vi "subvi_slope.vi"(1 "X1":dbl, 2 "X2":dbl, 3 "Y1":dbl, 4 "Y2":dbl) -> (0 "SLOPE":dbl)   [LabVIEW 2023]
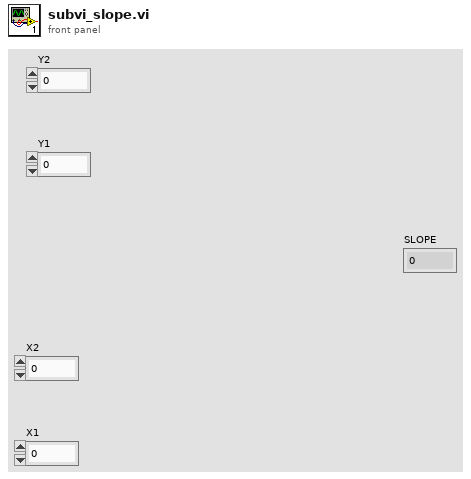
[diagram p1: front panel]
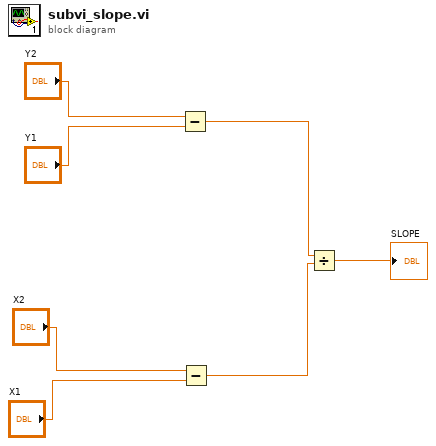
[diagram p0: block diagram]
diagram:
  n1 = Subtract(x="Y2", y="Y1") -> (x-y=w3:dbl)
  n2 = Subtract(x="X2", y="X1") -> (x-y=w2:dbl)
  n3 = Divide(x=w3, y=w2) -> (x/y=→"SLOPE":dbl)
